vi "曲线对齐-多曲线-XY图.vi"() -> ()   [LabVIEW 2015]
uses:
  <vilib>/Utility/miscctls.llb/LVCursorListTypeDef.ctl
  <vilib>/Utility/file.llb/Write Delimited Spreadsheet (string).vi
panel:
  in  "全部重采样":bool
  in  "删除所有":bool
  in  "Y数据":u16(ring) items=["数据1", "数据2"]
  in  "X数据":u16(ring) items=["数据1", "数据2"]
  in  "删除按钮":bool
  in  "添加按钮":bool
  out "XY图":cluster{"X":dbl, "Y":dbl}[](graph)
  out "数据名称":string[](array[string])
  in  "保存数据":bool
  in  "参考曲线":u16(ring) items=["数据1", "数据2", "无"]
  in  "编辑曲线":u16(ring) items=["数据1", "数据2"]
  in  "重采样间隔":dbl=0.1 min=1e-06 format="%.3fs"
  in  "取消修改":bool
  in  "确认修改":bool
  in  "功能选择":T1
  in  "加载数据":bool
  out "曲线对齐":cluster{"理论时间":dbl[], "力":dbl[]}[](graph)
  in  "测量曲线路径":path=path "D:/曲线处理/数据源.csv" caption="数据源"
  in  "Enqueue Element":bool caption="元素入队列"
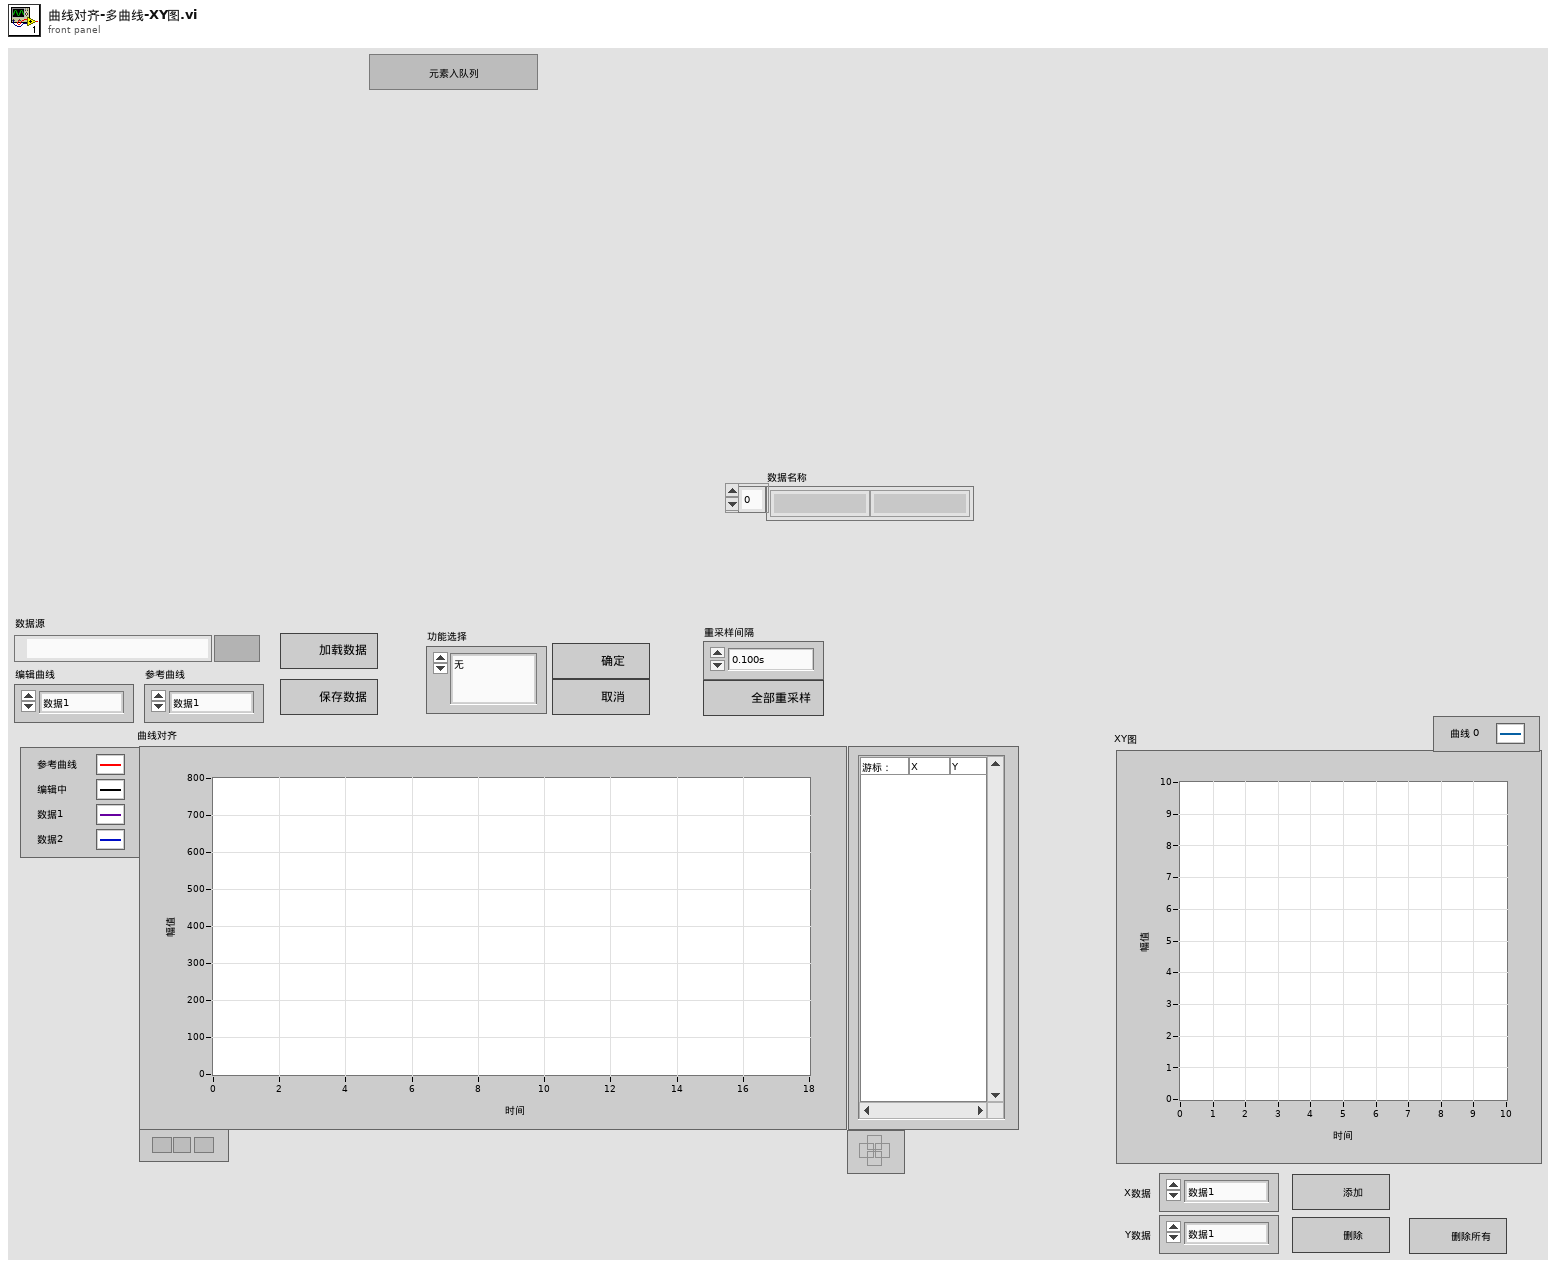
[diagram p1: front panel]
types:
  T1 = typedef "功能选择.ctl" = enum16{"无", "缩放曲线", "剪裁曲线", "对齐曲线", "初始值置0", "重采样", "曲线平滑"}
  T2 = typedef "曲线定义.ctl" = enum16{"编辑曲线", "参考曲线", "编辑中曲线"}
  T3 = typedef "LVCursorListTypeDef.ctl" = cluster{"Name":string, "Color":u32, "Style":u8, "Point Style":u8, "Name Visible":bool, "Allow Drag":bool, "Cursor Mode":u32, "Plot":i32, "Index":i32, "Position":cluster{"X":dbl, "Y":dbl}, "X Scale":u32, "Y Scale":u32, "Watch Plots":i32[], "Watch All Plots":bool, "Plot Area":i32, "Label Offset":cluster{"X":dbl, "Y":dbl}}[]
  T4 = cluster{"Name":string, "Color":u32, "Style":u8, "Point Style":u8, "Name Visible":bool, "Allow Drag":bool, "Cursor Mode":u32, "Plot":i32, "Index":i32, "Position":cluster{"X":dbl, "Y":dbl}, "X Scale":u32, "Y Scale":u32, "Watch Plots":i32[], "Watch All Plots":bool, "Plot Area":i32, "Label Offset":cluster{"X":dbl, "Y":dbl}}
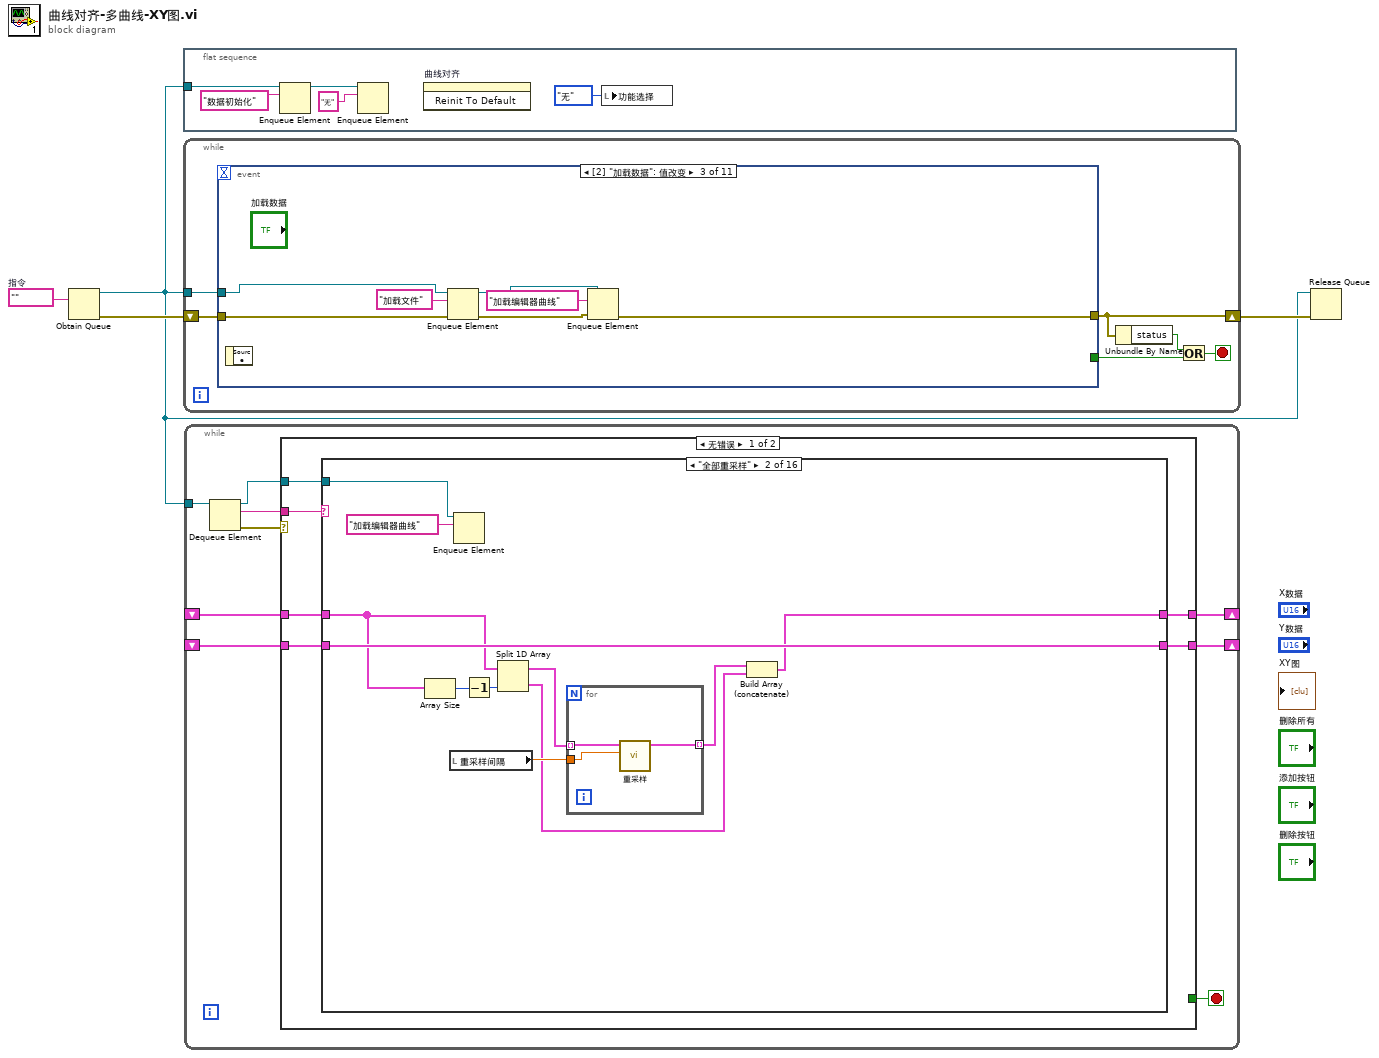
[diagram p0: block diagram]
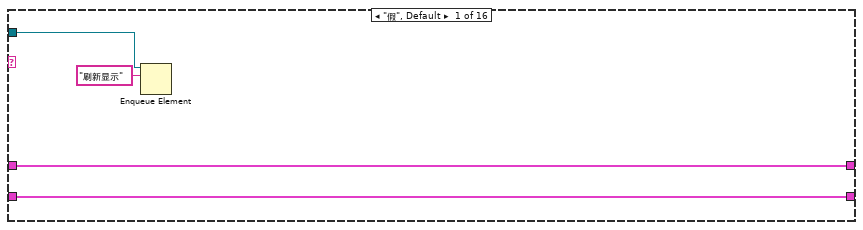
[diagram p2: hidden frame]
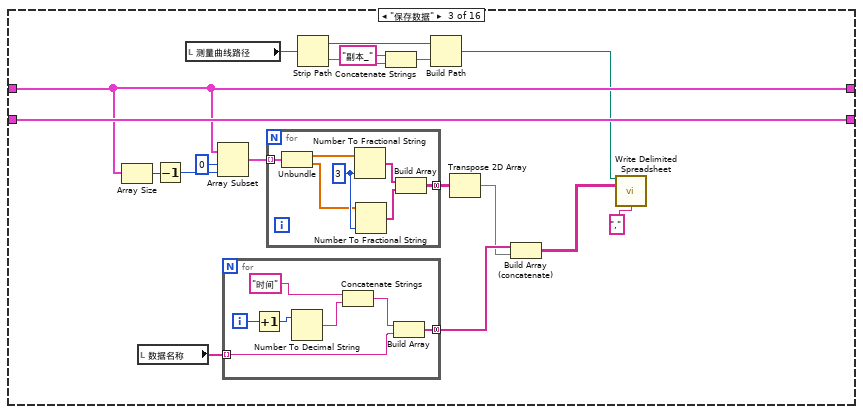
[diagram p3: hidden frame]
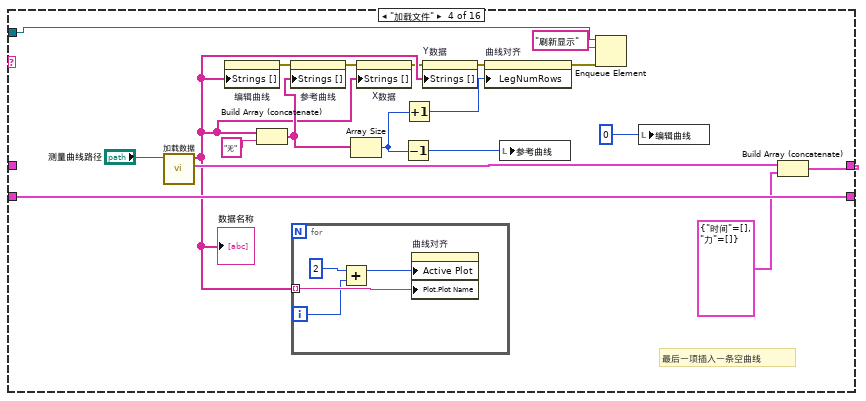
[diagram p4: hidden frame]
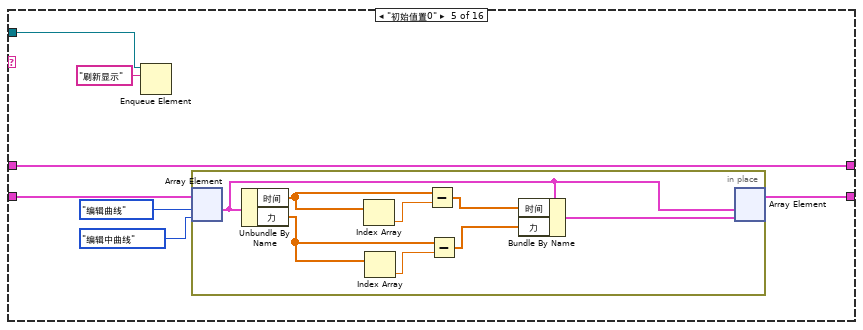
[diagram p5: hidden frame]
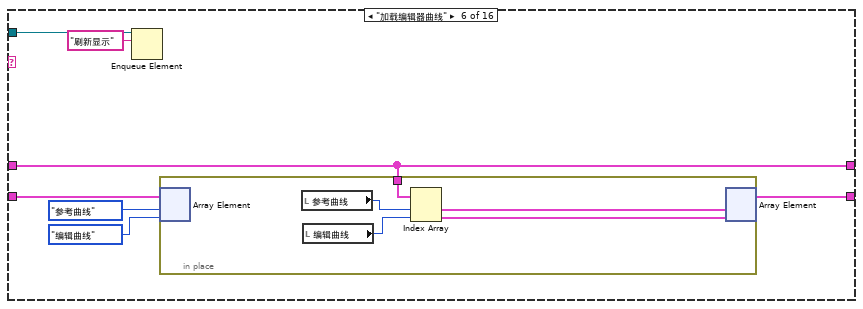
[diagram p6: hidden frame]
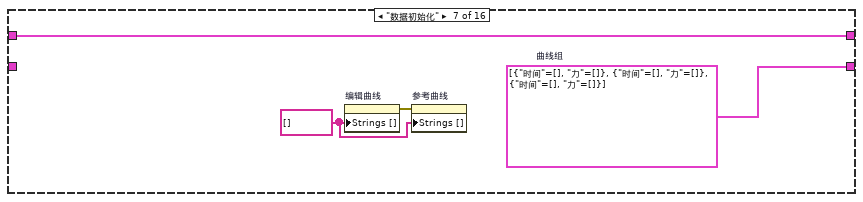
[diagram p7: hidden frame]
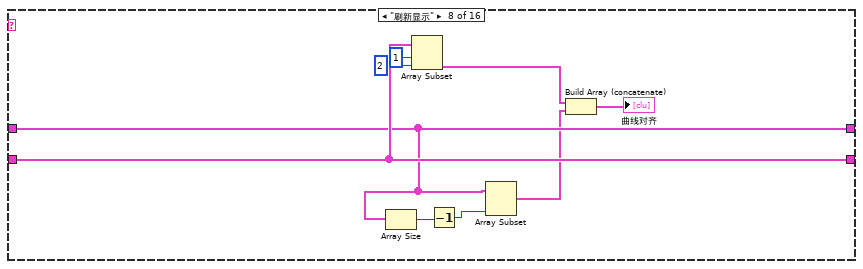
[diagram p8: hidden frame]
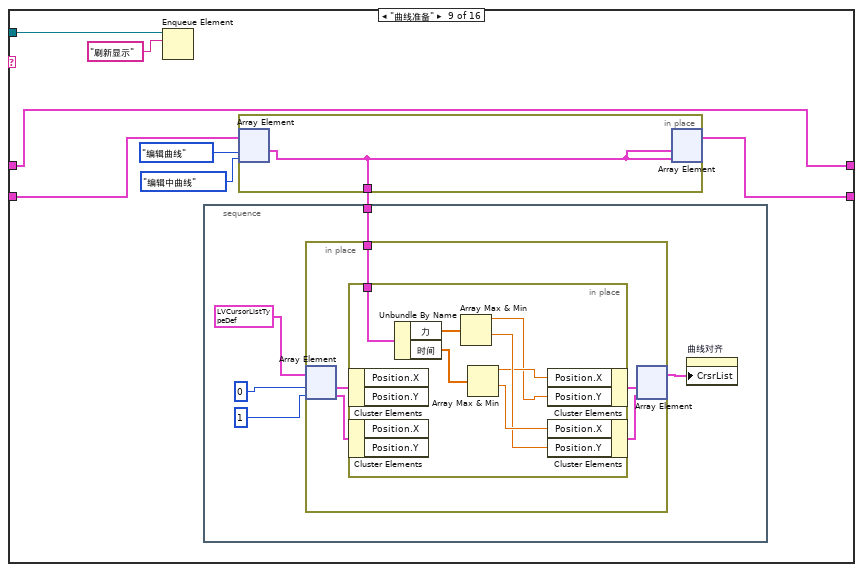
[diagram p9: hidden frame]
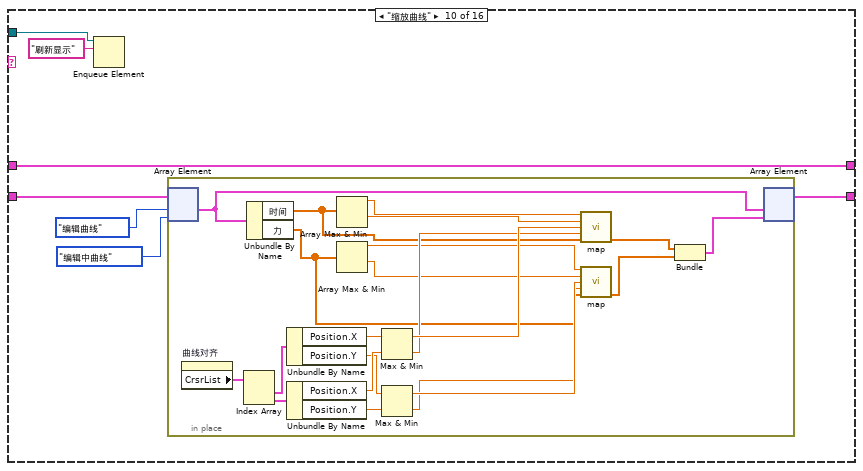
[diagram p10: hidden frame]
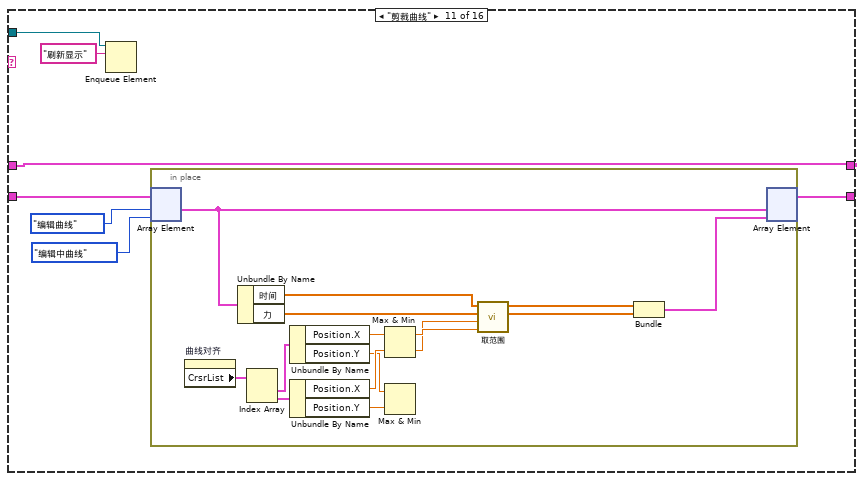
[diagram p11: hidden frame]
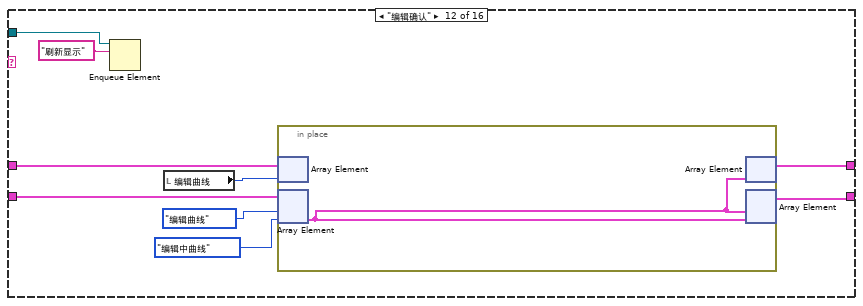
[diagram p12: hidden frame]
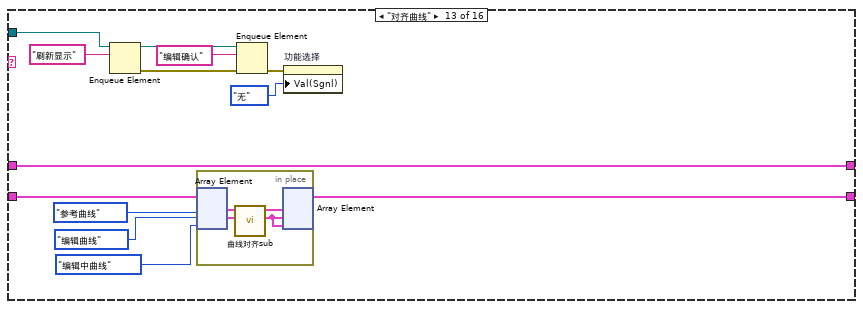
[diagram p13: hidden frame]
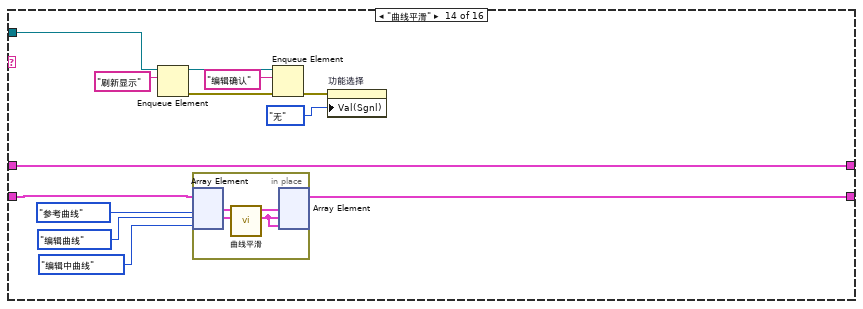
[diagram p14: hidden frame]
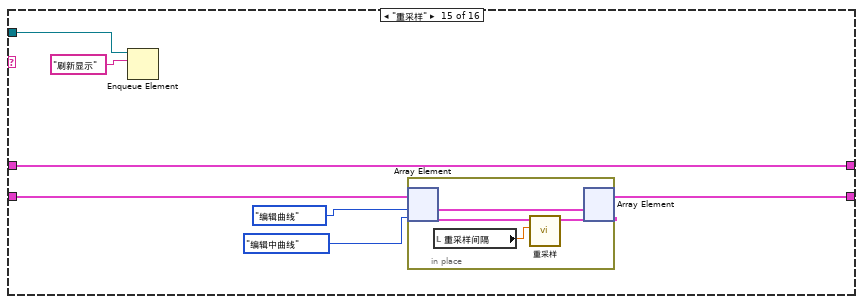
[diagram p15: hidden frame]
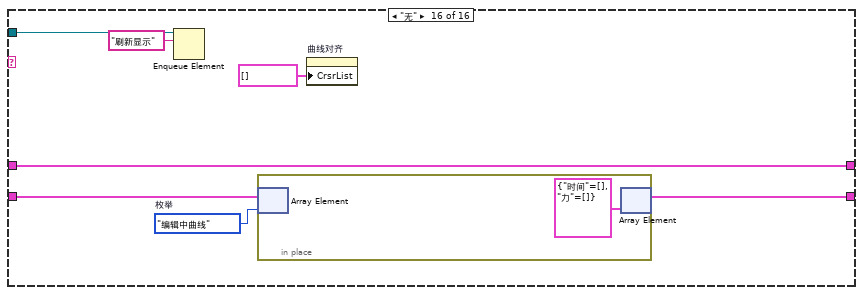
[diagram p16: hidden frame]
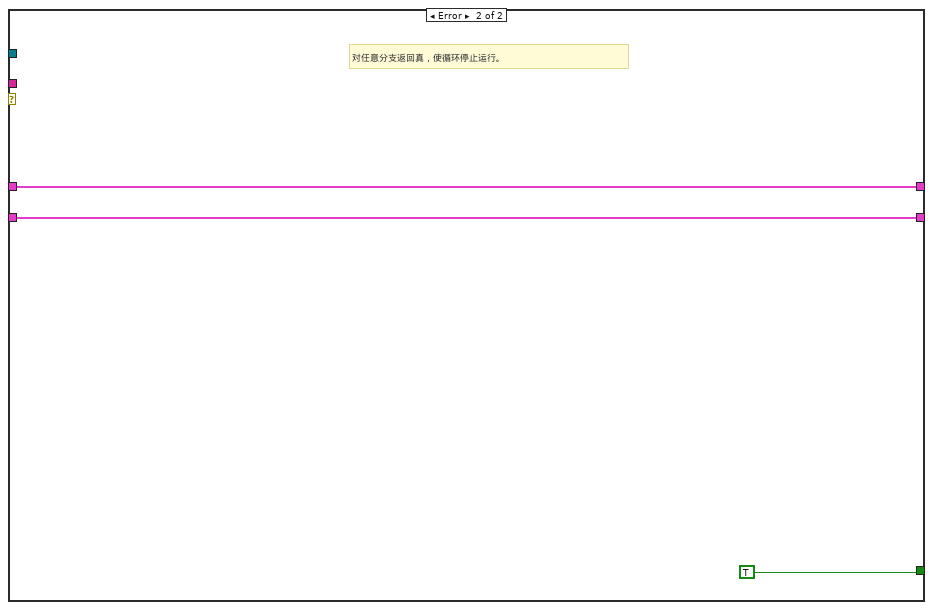
[diagram p17: hidden frame]
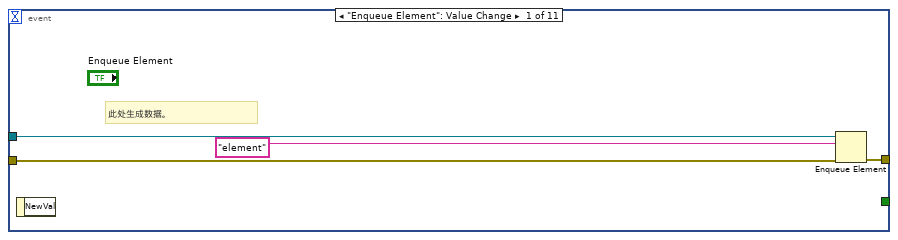
[diagram p18: hidden frame]
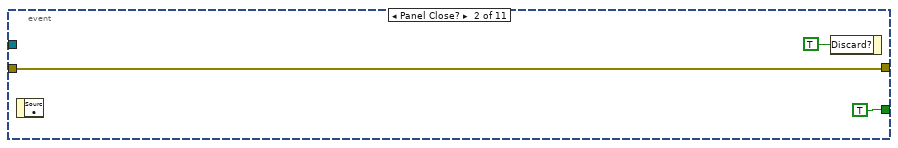
[diagram p19: hidden frame]
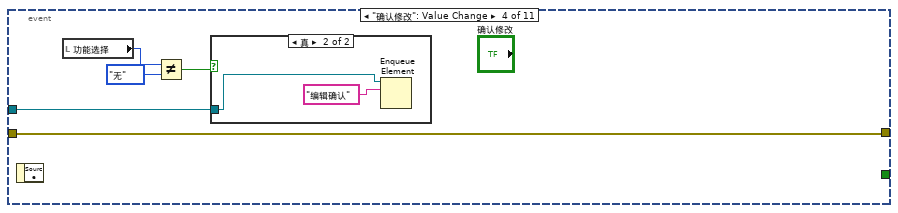
[diagram p20: hidden frame]
diagram:
  w4 = ""  # 指令
  n1 = Obtain Queue(element data type=w4) -> (queue out=w1:refnum<queue>, error out=w2:errorcluster)  [unwired: 4 in, 1 out]
  n2 = flat-sequence {
    tunnel: w1 -> [w8]
    frame #0 {
      n3 = Enqueue Element(queue=w8, element="数据初始化" ("元素")) -> (queue out=w6:refnum<queue>)  [unwired: 2 in, 2 out]
      n4 = Enqueue Element(queue=w6, element="无" ("元素")) -> ()  [unwired: 2 in, 3 out]
      n5 = invoke on="曲线对齐" class="XYGraph (严格)" method="Reinit To Default"() -> ()  [unwired: 3 in, 3 out]
      n6 = local write "功能选择"(功能选择."无" ("功能选择")) -> ()
    }
  }
  n7 = while {
    shift-right: [w11] -> w3
    shift-left: w2 -> [w14]
    tunnel: w1 -> [w15]
    stop <- w12 stop-if-true
    n8 = event shown="[2] \"加载数据\": 值改变" {
      selector: _ -> [_ _ _ _ _ _ _ _ _ _ _]
      dyn-events: _ -> [_ _ _ _ _ _ _ _ _ _ _]
      timeout: _ -> [_ _ _ _ _ _ _ _ _ _ _]
      tunnel: w15 -> [w19 _ w27 w33 _ w43 w49 w70 w72 w78 w80]
      tunnel: w14 -> [w18 w22 w26 w34 w38 w44 w51 w69 w74 w77 w82]
      tunnel: [w17 w22 w23 w34 w37 w44 w51 w66 w73 w76 w82] -> w11
      tunnel: [_ TRUE ("stop") _ _ _ _ _ _ _ _ _] -> w13
      event "Enqueue Element": Value Change {
        # "此处生成数据。"
        n9 = event-data() -> ()  [unwired: 1 in, 1 out]
        n10 = Enqueue Element(queue=w19, element="element", error in (no error)=w18) -> (error out=w17:errorcluster)  [unwired: 1 in, 2 out]
      }
      event Panel Close? {
        n11 = event-data() -> ()  [unwired: 1 in, 1 out]
        n12 = event-data("Discard?"=TRUE ("放弃？")) -> ()  [unwired: 1 in, 1 out]
      }
      event "加载数据": Value Change {
        n13 = event-data() -> ()  [unwired: 1 in, 1 out]
        n14 = Enqueue Element(queue=w27, element="加载文件" ("元素"), error in (no error)=w26) -> (queue out=w24:refnum<queue>, error out=w25:errorcluster)  [unwired: 1 in, 1 out]
        n15 = Enqueue Element(queue=w24, element="加载编辑器曲线" ("元素"), error in (no error)=w25) -> (error out=w23:errorcluster)  [unwired: 1 in, 2 out]
      }
      event "确认修改": Value Change {
        n16 = event-data() -> ()  [unwired: 1 in, 1 out]
        n17 = local read "功能选择"() -> (w32:T1)
        n18 = Not Equal?(x=w32, y=功能选择."无") -> (x != y?=w31:bool)
        n19 = case shown="真" w31 {
          tunnel: w33 -> [_ w35]
          frame False {
          }
          frame True {
            n20 = Enqueue Element(queue=w35, element="编辑确认" ("元素")) -> ()  [unwired: 2 in, 3 out]
          }
        }
      }
      event "取消修改": Value Change {
        n21 = event-data() -> ()  [unwired: 1 in, 1 out]
        n22 = property on="功能选择" class="Enum (严格)"(error in=w38, "Val(Sgnl)"=功能选择."无" ("值(信号)")) -> (error out=w37:errorcluster)  [unwired: 1 in, 1 out]
      }
      event "重采样间隔": Value Change {
        n23 = event-data() -> ()  [unwired: 1 in, 1 out]
        n24 = local read "功能选择"() -> (w41:T1)
        n25 = Equal?(x=w41, y=功能选择."重采样") -> (x = y?=w42:bool)
        n26 = case shown="真" w42 {
          tunnel: w43 -> [_ w45]
          frame False {
          }
          frame True {
            n27 = Enqueue Element(queue=w45, element="重采样" ("元素")) -> ()  [unwired: 2 in, 3 out]
          }
        }
      }
      event Value Change {
        n28 = event-data() -> ("NewVal"=w50:T1)  [unwired: 1 in]
        n29 = Enqueue Element(queue=w49, element="无" ("元素")) -> (queue out=w48:refnum<queue>)  [unwired: 2 in, 2 out]
        n30 = case shown="\"初始值置0\"" w50 {
          tunnel: w48 -> [w52 w55 w56 w58 w60 w63 w64]
          frame "缩放曲线", Default {
            n31 = Enqueue Element(queue=w52, element="曲线准备" ("元素")) -> ()  [unwired: 2 in, 3 out]
          }
          frame "无" {
            n32 = Enqueue Element(queue=w55, element="无" ("元素")) -> ()  [unwired: 2 in, 3 out]
          }
          frame "剪裁曲线" {
            n33 = Enqueue Element(queue=w56, element="曲线准备" ("元素")) -> ()  [unwired: 2 in, 3 out]
          }
          frame "对齐曲线" {
            n34 = Enqueue Element(queue=w58, element="对齐曲线" ("元素")) -> ()  [unwired: 2 in, 3 out]
          }
          frame "初始值置0" {
            n35 = Enqueue Element(queue=w60, element="初始值置0" ("元素")) -> ()  [unwired: 2 in, 3 out]
          }
          frame "重采样" {
            n36 = Enqueue Element(queue=w63, element="重采样" ("元素")) -> ()  [unwired: 2 in, 3 out]
          }
          frame "曲线平滑" {
            n37 = Enqueue Element(queue=w64, element="曲线平滑" ("元素")) -> ()  [unwired: 2 in, 3 out]
          }
        }
      }
      event "编辑曲线", "参考曲线": Value Change {
        n38 = event-data() -> ()  [unwired: 1 in, 1 out]
        n39 = Enqueue Element(queue=w70, element="加载编辑器曲线" ("元素"), error in (no error)=w69) -> (error out=w67:errorcluster)  [unwired: 1 in, 2 out]
        n40 = property on="功能选择" class="Enum (严格)"(error in=w67, "Val(Sgnl)"=功能选择."无" ("功能选择")) -> (error out=w66:errorcluster)  [unwired: 1 in, 1 out]
      }
      event "全部重采样": Value Change {
        n41 = event-data() -> ()  [unwired: 1 in, 1 out]
        n42 = Enqueue Element(queue=w72, element="全部重采样" ("元素"), error in (no error)=w74) -> (error out=w73:errorcluster)  [unwired: 1 in, 2 out]
      }
      event "保存数据": Value Change {
        n43 = event-data() -> ()  [unwired: 1 in, 2 out]
        n44 = Enqueue Element(queue=w78, element="保存数据" ("元素"), error in (no error)=w77) -> (error out=w76:errorcluster)  [unwired: 1 in, 2 out]
      }
      event "曲线对齐": Cursor Move {
        n45 = event-data() -> ()  [unwired: 1 in, 8 out]
        n46 = local read "功能选择"() -> (w81:T1)
        n47 = case shown="\"无\", 默认" w81 {
          tunnel: w80 -> [_ w83 w85]
          frame "无", Default {
          }
          frame "缩放曲线" {
            n48 = Enqueue Element(queue=w83, element="缩放曲线" ("元素")) -> ()  [unwired: 2 in, 3 out]
          }
          frame "剪裁曲线" {
            n49 = Enqueue Element(queue=w85, element="剪裁曲线" ("元素")) -> ()  [unwired: 2 in, 3 out]
          }
        }
      }
    }
    n50 = Unbundle By Name(w11) -> ("status"=w10:bool)
    n51 = Or(x=w10, y=w13) -> (x .or. y?=w12:bool)
  }
  n52 = while {
    tunnel: w1 -> [w90]
    shift-right: [w92] -> _
    shift-left: _ -> [w91]
    shift-right: [w88] -> _
    shift-left: _ -> [w87]
    stop <- w93 stop-if-true
    n53 = Dequeue Element(queue=w90) -> (queue out=w89:refnum<queue>, element=w94:string, error out=w95:errorcluster)  [unwired: 2 in, 1 out]
    n54 = case shown="无错误" w95 {
      tunnel: w94 -> [w101 _]
      tunnel: [_ TRUE] -> w93
      tunnel: [w98 w354] -> w92
      tunnel: w91 -> [w100 w354]
      tunnel: w89 -> [w99 _]
      tunnel: [w97 w353] -> w88
      tunnel: w87 -> [w96 w353]
      frame No Error {
        n55 = case shown="\"全部重采样\"" w101 {
          tunnel: [w103 w115 w136 w168 w179 w193 w205 w213 w218 w244 w272 w296 w310 w326 w338 w346] -> w98
          tunnel: w100 -> [w103 w115 w136 w168 w178 w194 _ w213 w219 w245 w273 w297 w309 w327 w339 w347]
          tunnel: w99 -> [w104 w116 _ w169 w180 w196 _ _ w221 w246 w274 w298 w312 w329 w340 w349]
          tunnel: [w102 w108 w132 w162 w175 w191 w204 w208 w215 w241 w269 w291 w305 w322 w335 w348] -> w97
          tunnel: w96 -> [w102 w112 w132 _ w175 w191 w204 w208 w215 w241 w269 w292 w305 w322 w335 w348]
          frame "假", Default {
            n56 = Enqueue Element(queue=w104, element="刷新显示" ("元素")) -> ()  [unwired: 2 in, 3 out]
          }
          frame "全部重采样" {
            n57 = Array Size(array=w112) -> (size(s)=w110:i32)
            n58 = local read "重采样间隔"() -> (w113:dbl)
            n59 = Enqueue Element(queue=w116, element="加载编辑器曲线" ("元素")) -> ()  [unwired: 2 in, 3 out]
            n60 = Decrement(x=w110) -> (x-1=w109:i32)
            n61 = Split 1D Array(array=w112, index=w109) -> (first subarray=w111:cluster{"时间":dbl[], "力":dbl[]}[], second subarray=w107:cluster{"时间":dbl[], "力":dbl[]}[])
            n62 = for {
              tunnel: w111 -> [w119] mode=indexing
              tunnel: [w118] -> w114 mode=indexing
              tunnel: w113 -> [w117]
              n63 = call "重采样.vi"("重采样间隔"=w117, "输出簇"=w119) -> ("簇"=w118:cluster{"xi used":dbl[], "yi":dbl[]})  [unwired: 9 in]
            }
            n64 = Build Array (concatenate)(w114, w107) -> (w108:cluster{"时间":dbl[], "力":dbl[]}[])
          }
          frame "保存数据" {
            n65 = Array Size(array=w132) -> (size(s)=w137:i32)
            n66 = local read "数据名称"() -> (w123:string[])
            n67 = Decrement(x=w137) -> (x-1=w135:i32)
            n68 = local read "测量曲线路径"() -> (w131:path)
            n69 = Array Subset(array=w132, index=0 ("索引"), length=w135) -> (w134:cluster{"时间":dbl[], "力":dbl[]}[])
            n70 = for {
              tunnel: w123 -> [w139] mode=indexing
              tunnel: [w138] -> w122 mode=concatenating
              i -> [w144]
              n71 = Increment(x=w144) -> (x+1=w143:i32)
              n72 = Number To Decimal String(number=w143) -> (decimal integer string=w141:string)  [unwired: 1 in]
              n73 = Concatenate Strings("时间", w141) -> (w140:string)
              n74 = Build Array(w140, w139) -> (w138:string[])
            }
            n75 = for {
              tunnel: w134 -> [w151] mode=indexing
              tunnel: [w145] -> w124 mode=concatenating
              w150 = i16 3 ("精度(6)")
              n76 = Unbundle(w151) -> ("时间"=w149:dbl[], "力"=w148:dbl[])
              n77 = Number To Fractional String(number=w149, precision (6)=w150) -> (F-format string=w147:string[])  [unwired: 2 in]
              n78 = Number To Fractional String(number=w148, precision (6)=w150) -> (F-format string=w146:string[])  [unwired: 2 in]
              n79 = Build Array(w147, w146) -> (w145:string[][])
            }
            n80 = Strip Path(path=w131) -> (stripped path=w130:path, name=w129:string)
            n81 = Concatenate Strings("副本_" ("字符串"), w129) -> (w127:string)
            n82 = Build Path(base path=w130, name or relative path=w127) -> (appended path=w126:path)
            n83 = Transpose 2D Array(2D array=w124) -> (transposed array=w121:string[][])
            n84 = Build Array (concatenate)(w122, w121) -> (w120:string[][])
            n85 = call-poly <vilib>:"Write Delimited Spreadsheet.vi"("file path (dialog if empty)"=w126, "2D data"=w120, "delimiter (\\t)"="," ("delimiter (\\t)")) -> ()  [unwired: 11 in, 2 out]
          }
          frame "加载文件" {
            # "最后一项插入一条空曲线"
            n86 = call "加载数据.vi"("数据路径"="测量曲线路径") -> ("数据"=w166:cluster{dbl[], dbl[]}[], "数据名称"=w156:string[])  [unwired: 9 in]
            "数据名称" <- w156
            n87 = property on="编辑曲线" class="Ring (严格)"("Strings []"=w156) -> (error out=w164:errorcluster)  [unwired: 2 in, 1 out]
            n88 = Build Array (concatenate)(w156, "无") -> (w159:string[])
            n89 = property on="参考曲线" class="Ring (严格)"(error in=w164, "Strings []"=w159) -> (error out=w155:errorcluster)  [unwired: 1 in, 1 out]
            n90 = for {
              tunnel: w156 -> [w174] mode=indexing
              i -> [w173]
              n91 = Add(x=2 ("y"), y=w173) -> (x+y=w172:i32)
              n92 = property on="曲线对齐" class="XYGraph (严格)"("Active Plot"=w172, "Plot.Plot Name"=w174) -> ()  [unwired: 2 in, 2 out]
            }
            n93 = Array Size(array=w159) -> (size(s)=w157:i32)
            n94 = property on="X数据" class="Ring (严格)"(error in=w155, "Strings []"=w156) -> (error out=w154:errorcluster)  [unwired: 1 in, 1 out]
            n95 = Decrement(x=w157) -> (x-1=w160:i32)
            n96 = Increment(x=w157) -> (x+1=w158:i32)
            n97 = property on="Y数据" class="Ring (严格)"(error in=w154, "Strings []"=w156) -> (error out=w153:errorcluster)  [unwired: 1 in, 1 out]
            n98 = property on="曲线对齐" class="XYGraph (严格)"(error in=w153, "LegNumRows"=w158) -> (error out=w152:errorcluster)  [unwired: 1 in, 1 out]
            n99 = local write "参考曲线"(w160) -> ()
            n100 = Enqueue Element(queue=w169, element="刷新显示" ("元素"), error in (no error)=w152) -> ()  [unwired: 1 in, 3 out]
            n101 = local write "编辑曲线"(0) -> ()
            n102 = Build Array (concatenate)(w166, cluster{"时间":dbl[], "力":dbl[]} {"时间"=[], "力"=[]} ("输出簇")) -> (w162:cluster{"时间":dbl[], "力":dbl[]}[])
          }
          frame "初始值置0" {
            n103 = Enqueue Element(queue=w180, element="刷新显示" ("元素")) -> ()  [unwired: 2 in, 3 out]
            n104 = in-place {
              n105 = in-place-array #1(w178, 曲线定义."编辑曲线", 曲线定义."编辑中曲线") -> (w183:cluster{"时间":dbl[], "力":dbl[]})  [unwired: 1 out]
              n106 = Unbundle By Name(w183) -> ("时间"=w189:dbl[], "力"=w187:dbl[])
              n107 = Index Array(array=w189) -> (element=w188:dbl)  [unwired: 1 in]
              n108 = Index Array(array=w187) -> (element=w186:dbl)  [unwired: 1 in]
              n109 = Subtract(x=w189, y=w188) -> (x-y=w185:dbl[])
              n110 = Subtract(x=w187, y=w186) -> (x-y=w184:dbl[])
              n111 = Bundle By Name(cluster=w183, "时间"=w185, "力"=w184) -> (w182:cluster{"时间":dbl[], "力":dbl[]})
              n112 = in-place-array #1(w183, w182) -> (w179:cluster{"时间":dbl[], "力":dbl[]}[])  [unwired: 2 out]
            }
          }
          frame "加载编辑器曲线" {
            n113 = Enqueue Element(queue=w196, element="刷新显示" ("元素")) -> ()  [unwired: 2 in, 3 out]
            n114 = in-place {
              in-place-border: w191 -> [w201]
              n115 = in-place-array #2(w194, 曲线定义."参考曲线", 曲线定义."编辑曲线") -> ()  [unwired: 2 out]
              n116 = local read "参考曲线"() -> (w198:u16)
              n117 = local read "编辑曲线"() -> (w199:u16)
              n118 = Index Array(array=w201, index #1=w198, index #2=w199) -> (element #1=w197:cluster{"时间":dbl[], "力":dbl[]}, element #2=w200:cluster{"时间":dbl[], "力":dbl[]})
              n119 = in-place-array #2(w197, w200) -> (w193:cluster{"时间":dbl[], "力":dbl[]}[])  [unwired: 2 out]
            }
          }
          frame "数据初始化" {
            w203 = string[] [] ("字符串[]")
            w205 = cluster{"时间":dbl[], "力":dbl[]}[] [{"时间"=[], "力"=[]}, {"时间"=[], "力"=[]}, {"时间"=[], "力"=[]}]  # 曲线组
            n120 = property on="编辑曲线" class="Ring (严格)"("Strings []"=w203) -> (error out=w202:errorcluster)  [unwired: 2 in, 1 out]
            n121 = property on="参考曲线" class="Ring (严格)"(error in=w202, "Strings []"=w203) -> ()  [unwired: 1 in, 2 out]
          }
          frame "刷新显示" {
            n122 = Array Size(array=w208) -> (size(s)=w209:i32)
            n123 = Array Subset(array=w213, index=1 ("索引"), length=2 ("长度")) -> (w210:cluster{"时间":dbl[], "力":dbl[]}[])
            n124 = Decrement(x=w209) -> (x-1=w207:i32)
            n125 = Array Subset(array=w208, length=w207) -> (w206:cluster{"时间":dbl[], "力":dbl[]}[])  [unwired: 1 in]
            n126 = Build Array (concatenate)(w210, w206) -> (→"曲线对齐":cluster{"时间":dbl[], "力":dbl[]}[])
          }
          frame "曲线准备" {
            n127 = Enqueue Element(queue=w221, element="刷新显示" ("元素")) -> ()  [unwired: 2 in, 3 out]
            n128 = in-place {
              in-place-border: [w223] -> w220
              n129 = in-place-array #3(w219, 曲线定义."编辑曲线", 曲线定义."编辑中曲线") -> (w223:cluster{"时间":dbl[], "力":dbl[]})  [unwired: 1 out]
              n130 = in-place-array #3(w223, w223) -> (w218:cluster{"时间":dbl[], "力":dbl[]}[])  [unwired: 2 out]
            }
            n131 = stacked-sequence {
              tunnel: w220 -> [w224]
              frame #0 {
                n132 = in-place {
                  in-place-border: w224 -> [w229]
                  n133 = in-place-array #4(T3 [{"Name"="游标0", "Color"=16711680, "Style"=8, "Point Style"=13, "Name Visible"=FALSE, "Allow Drag"=TRUE, "Cursor Mode"=0, "Plot"=0, "Index"=0, "Position"={"X"=24.900169204737733, "Y"=876.3513513513514}, "X Scale"=0, "Y Scale"=0, "Watch Plots"=[], "Watch All Plots"=FALSE, "Plot Area"=0, "Label Offset"={"X"=0.0, "Y"=67.56756756756761}}, {"Name"="游标1", "Color"=16860, "Style"=8, "Point Style"=13, "Name Visible"=FALSE, "Allow Drag"=TRUE, "Cursor Mode"=0, "Plot"=0, "Index"=0, "Position"={"X"=-2.199661590524536, "Y"=1.3513513513513553}, "X Scale"=0, "Y Scale"=0, "Watch Plots"=[], "Watch All Plots"=FALSE, "Plot Area"=0, "Label Offset"={"X"=8.881784197001252e-16, "Y"=67.56756756756756}}] ("游标列表"), 0, 1) -> (w233:T4, w232:T4)
                  n134 = in-place {
                    in-place-border: w229 -> [w236]
                    n135 = in-place-cluster #5(w233) -> ()  [unwired: 2 out]
                    n136 = in-place-cluster #6(w232) -> ()  [unwired: 2 out]
                    n137 = Unbundle By Name(w236) -> ("力"=w235:dbl[], "时间"=w234:dbl[])
                    n138 = Array Max & Min(array=w235) -> (max value=w237:dbl, min value=w239:dbl)  [unwired: 2 out]
                    n139 = Array Max & Min(array=w234) -> (max value=w238:dbl, min value=w240:dbl)  [unwired: 2 out]
                    n140 = in-place-cluster #5("Position.X"=w238, "Position.Y"=w237) -> (w231:T4)
                    n141 = in-place-cluster #6("Position.X"=w240, "Position.Y"=w239) -> (w230:T4)
                  }
                  n142 = in-place-array #4(w231, w230) -> (w225:T3)  [unwired: 2 out]
                }
                n143 = property on="曲线对齐" class="XYGraph (严格)"("CrsrList"=w225) -> ()  [unwired: 2 in, 2 out]
              }
            }
          }
          frame "缩放曲线" {
            n144 = Enqueue Element(queue=w246, element="刷新显示" ("元素")) -> ()  [unwired: 2 in, 3 out]
            n145 = in-place {
              n146 = in-place-array #7(w245, 曲线定义."编辑曲线", 曲线定义."编辑中曲线") -> (w250:cluster{"时间":dbl[], "力":dbl[]})  [unwired: 1 out]
              n147 = property on="曲线对齐" class="XYGraph (严格)"() -> ("CrsrList"=w268:T3)  [unwired: 2 in, 2 out]
              n148 = Index Array(array=w268) -> (element #1=w267:T4, element #2=w266:T4)  [unwired: 2 in]
              n149 = Unbundle By Name(w250) -> ("时间"=w249:dbl[], "力"=w248:dbl[])
              n150 = Unbundle By Name(w267) -> ("Position.X"=w265:dbl, "Position.Y"=w263:dbl)
              n151 = Unbundle By Name(w266) -> ("Position.X"=w264:dbl, "Position.Y"=w262:dbl)
              n152 = Array Max & Min(array=w249) -> (max value=w261:dbl, min value=w260:dbl)  [unwired: 2 out]
              n153 = Array Max & Min(array=w248) -> (max value=w257:dbl, min value=w256:dbl)  [unwired: 2 out]
              n154 = Max & Min(x=w265, y=w264) -> (max(x,y)=w259:dbl, min(x,y)=w258:dbl)
              n155 = Max & Min(x=w263, y=w262) -> (max(x,y)=w255:dbl, min(x,y)=w254:dbl)
              n156 = call "map.vi"("inmax"=w261, "inmin"=w260, "outmax"=w259, "outmin"=w258, "in"=w249) -> ("out"=w253:dbl[])  [unwired: 10 in]
              n157 = call "map.vi"("inmax"=w257, "inmin"=w256, "outmax"=w255, "outmin"=w254, "in"=w248) -> ("out"=w252:dbl[])  [unwired: 10 in]
              n158 = Bundle("out"=w253, "out"=w252) -> (w251:cluster{"out":dbl[], "out":dbl[]})  [unwired: 1 in]
              n159 = in-place-array #7(w250, w251) -> (w244:cluster{"时间":dbl[], "力":dbl[]}[])  [unwired: 2 out]
            }
          }
          frame "剪裁曲线" {
            n160 = Enqueue Element(queue=w274, element="刷新显示" ("元素")) -> ()  [unwired: 2 in, 3 out]
            n161 = in-place {
              n162 = in-place-array #8(w273, 曲线定义."编辑曲线", 曲线定义."编辑中曲线") -> (w283:cluster{"时间":dbl[], "力":dbl[]})  [unwired: 1 out]
              n163 = property on="曲线对齐" class="XYGraph (严格)"() -> ("CrsrList"=w290:T3)  [unwired: 2 in, 2 out]
              n164 = Unbundle By Name(w283) -> ("时间"=w280:dbl[], "力"=w279:dbl[])
              n165 = Index Array(array=w290) -> (element #1=w289:T4, element #2=w288:T4)  [unwired: 2 in]
              n166 = Unbundle By Name(w289) -> ("Position.X"=w287:dbl, "Position.Y"=w285:dbl)
              n167 = Unbundle By Name(w288) -> ("Position.X"=w286:dbl, "Position.Y"=w284:dbl)
              n168 = Max & Min(x=w287, y=w286) -> (max(x,y)=w282:dbl, min(x,y)=w281:dbl)
              n169 = Max & Min(x=w285, y=w284) -> ()  [unwired: 2 out]
              n170 = call "取范围.vi"("max"=w282, "min"=w281, "y"=w279, "x"=w280) -> ("y"=w277:dbl[], "x"=w278:dbl[])  [unwired: 6 in]
              n171 = Bundle("x"=w278, "y"=w277) -> (w276:cluster{"x":dbl[], "y":dbl[]})  [unwired: 1 in]
              n172 = in-place-array #8(w283, w276) -> (w272:cluster{"时间":dbl[], "力":dbl[]}[])  [unwired: 2 out]
            }
          }
          frame "编辑确认" {
            n173 = Enqueue Element(queue=w298, element="刷新显示" ("元素")) -> ()  [unwired: 2 in, 3 out]
            n174 = local read "编辑曲线"() -> (w293:u16)
            n175 = in-place {
              n176 = in-place-array #9(w292, w293) -> ()  [unwired: 1 out]
              n177 = in-place-array #10(w297, 曲线定义."编辑曲线", 曲线定义."编辑中曲线") -> (w300:cluster{"时间":dbl[], "力":dbl[]})  [unwired: 1 out]
              n178 = in-place-array #9(w300) -> (w291:cluster{"时间":dbl[], "力":dbl[]}[])  [unwired: 1 out]
              n179 = in-place-array #10(w300, w300) -> (w296:cluster{"时间":dbl[], "力":dbl[]}[])  [unwired: 2 out]
            }
          }
          frame "对齐曲线" {
            n180 = Enqueue Element(queue=w312, element="刷新显示" ("元素")) -> (queue out=w303:refnum<queue>, error out=w301:errorcluster)  [unwired: 2 in, 1 out]
            n181 = in-place {
              n182 = in-place-array #11(w309, 曲线定义."参考曲线", 曲线定义."编辑曲线", 曲线定义."编辑中曲线") -> (w317:cluster{"时间":dbl[], "力":dbl[]}, w316:cluster{"时间":dbl[], "力":dbl[]})  [unwired: 1 out]
              n183 = call "曲线对齐sub.vi"("测量"=w316, "理论"=w317) -> ("实测"=w314:cluster{dbl[], dbl[]}, "理论"=w315:cluster{dbl[], dbl[]})  [unwired: 8 in]
              n184 = in-place-array #11(w315, w314, w314) -> (w310:cluster{"时间":dbl[], "力":dbl[]}[])  [unwired: 3 out]
            }
            n185 = Enqueue Element(queue=w303, element="编辑确认" ("元素"), error in (no error)=w301) -> (error out=w302:errorcluster)  [unwired: 1 in, 2 out]
            n186 = property on="功能选择" class="Enum (严格)"(error in=w302, "Val(Sgnl)"=功能选择."无" ("功能选择")) -> ()  [unwired: 1 in, 2 out]
          }
          frame "曲线平滑" {
            n187 = Enqueue Element(queue=w329, element="刷新显示" ("元素")) -> (queue out=w320:refnum<queue>, error out=w319:errorcluster)  [unwired: 2 in, 1 out]
            n188 = in-place {
              n189 = in-place-array #12(w327, 曲线定义."参考曲线", 曲线定义."编辑曲线", 曲线定义."编辑中曲线") -> (w334:cluster{"时间":dbl[], "力":dbl[]}, w333:cluster{"时间":dbl[], "力":dbl[]})  [unwired: 1 out]
              n190 = call "曲线平滑.vi"("测量"=w333, "理论"=w334) -> ("实测"=w331:cluster{dbl[], dbl[]}, "理论"=w332:cluster{dbl[], dbl[]})  [unwired: 8 in]
              n191 = in-place-array #12(w332, w331, w331) -> (w326:cluster{"时间":dbl[], "力":dbl[]}[])  [unwired: 3 out]
            }
            n192 = Enqueue Element(queue=w320, element="编辑确认" ("元素"), error in (no error)=w319) -> (error out=w318:errorcluster)  [unwired: 1 in, 2 out]
            n193 = property on="功能选择" class="Enum (严格)"(error in=w318, "Val(Sgnl)"=功能选择."无" ("功能选择")) -> ()  [unwired: 1 in, 2 out]
          }
          frame "重采样" {
            n194 = Enqueue Element(queue=w340, element="刷新显示" ("元素")) -> ()  [unwired: 2 in, 3 out]
            n195 = in-place {
              n196 = in-place-array #13(w339, 曲线定义."编辑曲线", 曲线定义."编辑中曲线") -> (w343:cluster{"时间":dbl[], "力":dbl[]})  [unwired: 1 out]
              n197 = local read "重采样间隔"() -> (w342:dbl)
              n198 = call "重采样.vi"("重采样间隔"=w342, "输出簇"=w343) -> ("簇"=w344:cluster{"xi used":dbl[], "yi":dbl[]})  [unwired: 9 in]
              n199 = in-place-array #13(w343, w344) -> (w338:cluster{"时间":dbl[], "力":dbl[]}[])  [unwired: 2 out]
            }
          }
          frame "无" {
            w345 = 曲线定义."编辑中曲线"  # 枚举
            n200 = Enqueue Element(queue=w349, element="刷新显示" ("元素")) -> ()  [unwired: 2 in, 3 out]
            n201 = in-place {
              n202 = in-place-array #14(w347, w345) -> ()  [unwired: 1 out]
              n203 = in-place-array #14(cluster{"时间":dbl[], "力":dbl[]} {"时间"=[], "力"=[]} ("元素")) -> (w346:cluster{"时间":dbl[], "力":dbl[]}[])  [unwired: 1 out]
            }
            n204 = property on="曲线对齐" class="XYGraph (严格)"("CrsrList"=T3 [] ("游标列表")) -> ()  [unwired: 2 in, 2 out]
          }
        }
      }
      frame Error {
        # "对任意分支返回真，使循环停止运行。"
      }
    }
  }
  n205 = Release Queue(queue=w1, error in (no error)=w3) -> ()  [unwired: 1 in, 3 out]
